vi "Coding table.vi"(10 "Bcd":u8) -> (0 "Alarm":string, 1 "Distance":i32, 2 "StepE":i32, 3 "StepM":i32)   [LabVIEW 2017]
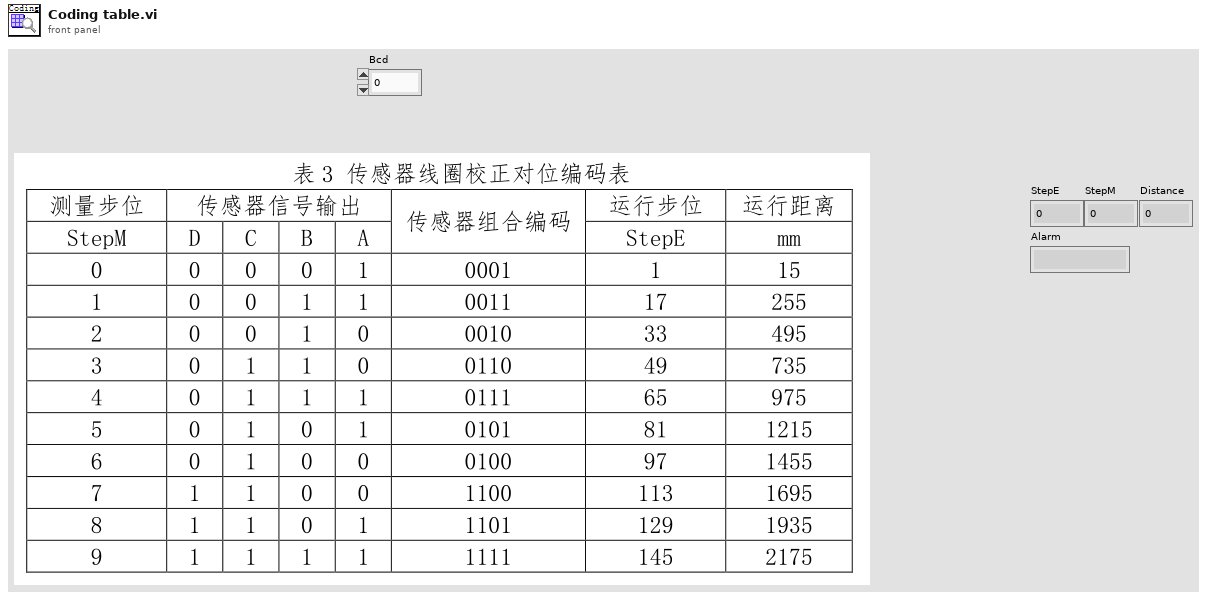
[diagram p1: front panel]
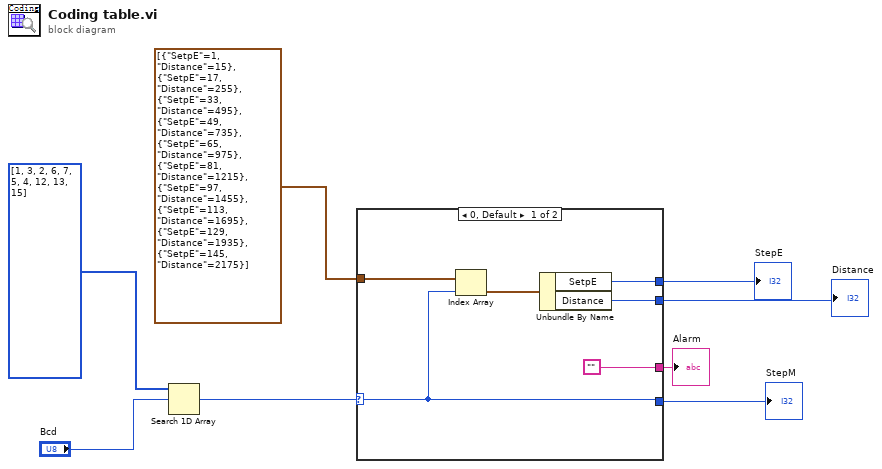
[diagram p0: block diagram]
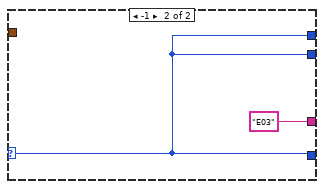
[diagram p2: hidden frame]
diagram:
  n1 = Search 1D Array(1D array=u8[] [1, 3, 2, 6, 7, 5, 4, 12, 13, 15] ("sencer code"), element="Bcd") -> (index of element=w6:i32)  [unwired: 1 in]
  n2 = case shown="0, Default" w6 {
    selector: w6 -> [w10 w16]
    tunnel: cluster{"SetpE":i32, "Distance":i32}[] [{"SetpE"=1, "Distance"=15}, {"SetpE"=17, "Distance"=255}, {"SetpE"=33, "Distance"=495}, {"SetpE"=49, "Distance"=735}, {"SetpE"=65, "Distance"=975}, {"SetpE"=81, "Distance"=1215}, {"SetpE"=97, "Distance"=1455}, {"SetpE"=113, "Distance"=1695}, {"SetpE"=129, "Distance"=1935}, {"SetpE"=145, "Distance"=2175}] -> [w14 _]
    tunnel: [w12 w16] -> w4
    tunnel: [w11 w16] -> w1
    tunnel: [w10 w16] -> w3
    tunnel: ["" "E03"] -> w2
    frame 0, Default {
      n3 = Index Array(array=w14, index=w10) -> (element=w13:cluster{"SetpE":i32, "Distance":i32})
      n4 = Unbundle By Name(w13) -> ("SetpE"=w12:i32, "Distance"=w11:i32)
    }
    frame -1 {
    }
  }
  "StepE" <- w4
  "StepM" <- w3
  "Alarm" <- w2
  "Distance" <- w1
